vi "WhichClicked.vi"(0 "Buttons":bool[][](array[boolean])) -> (1 "X":i32, 2 "Y":i32, 3 "OneClicked?":bool)   [LabVIEW 2018]
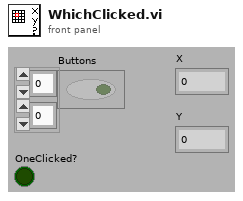
[diagram p1: front panel]
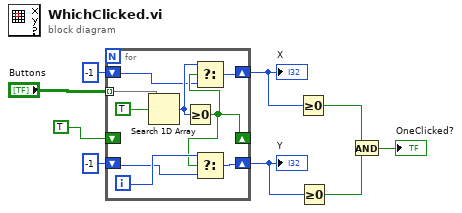
[diagram p0: block diagram]
diagram:
  n1 = for {
    tunnel: "Buttons" -> [w18] mode=indexing
    shift-right: [w13] -> _
    shift-left: TRUE -> [_]
    shift-right: [w16] -> w4
    shift-left: -1 -> [w14]
    shift-right: [w10] -> w5
    shift-left: -1 ("index of element") -> [w11]
    i -> [w15]
    n2 = Search 1D Array(1D array=w18, element=TRUE) -> (index of element=w12:i32)  [unwired: 1 in]
    n3 = Greater Or Equal To 0?(x=w12) -> (x >= 0?=w13:bool)
    n4 = Select(t=w12, s=w13, f=w11) -> (s? t:f=w10:i32)
    n5 = Select(t=w15, s=w13, f=w14) -> (s? t:f=w16:i32)
  }
  "Y" <- w4
  "X" <- w5
  n6 = Greater Or Equal To 0?(x=w5) -> (x >= 0?=w2:bool)
  n7 = Greater Or Equal To 0?(x=w4) -> (x >= 0?=w3:bool)
  n8 = And(x=w2, y=w3) -> (x .and. y?=→"OneClicked?":bool)
